vi "Check_Needed_Files.vi"(3 "error in":errorcluster, 6 "Data Cluster":T1 {"Shaft"."dmin" format="%#_7g"; "Shaft"."dmax" format="%#_7g"; "Shaft"."Fundamental Dev" format="%#_7g"; "Shaft"."Tolerance Grade (IT) Shaft" format="%#_7g"; "Hole"."Dmin" format="%#_7g"; "Hole"."Tolerance Grade (IT)" format="%#_7g"}) -> (0 "error out 2":errorcluster)   [LabVIEW 2023]
uses:
  TypeDef/Data_Cluster.ctl
  <vilib>/MGI/Panel Manager/Panel/Panel/Window/Window.lvclass
  C:/Program Files (x86)/National Instruments/LabVIEW 2023/vi.lib/MGI/Panel Manager/Panel/Panel/Panel.lvclass
  TypeDef/Units.ctl
  TypeDef/Method_Info.ctl
  TypeDef/Hole_Data.ctl
  TypeDef/Shaft_Data.ctl
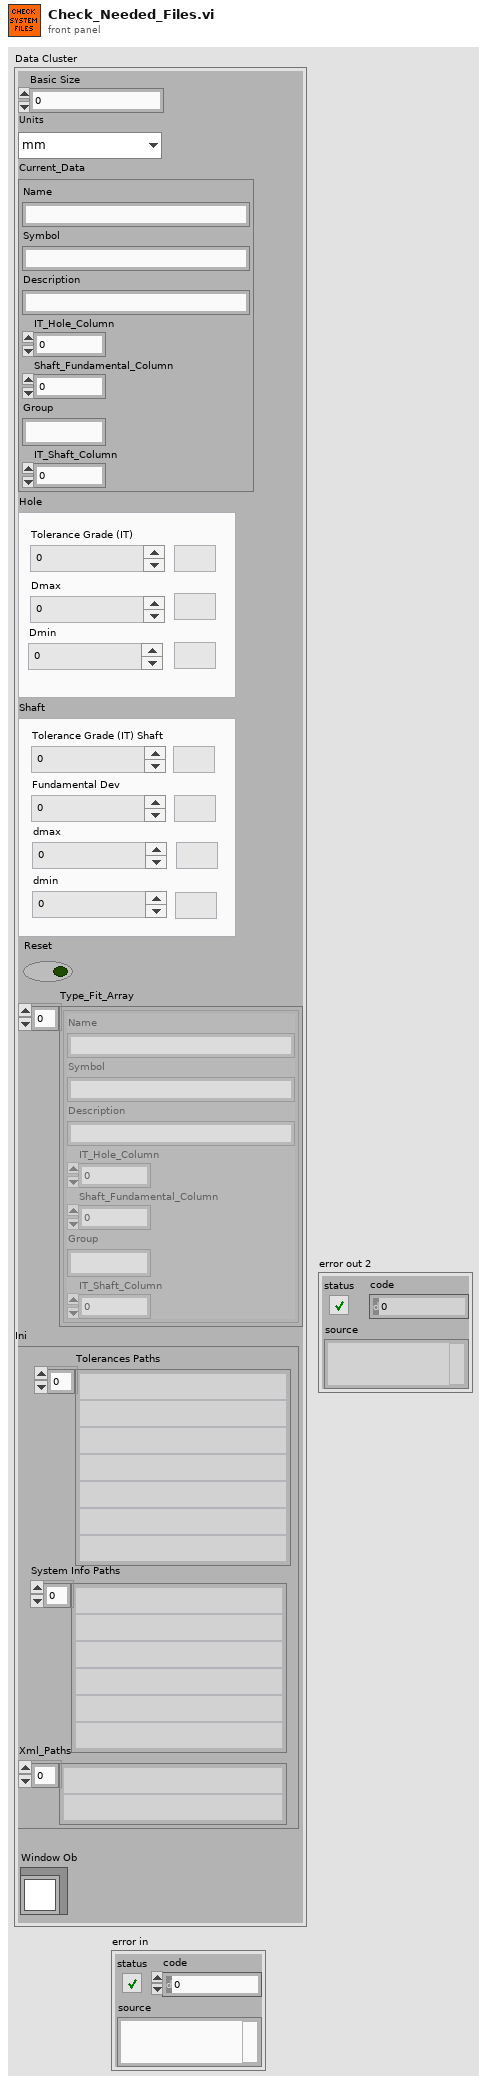
[diagram p1: front panel]
types:
  T1 = typedef "Data_Cluster.ctl" = cluster{"Basic Size ":dbl, "Units":T2, "Current_Data":T3, "Hole":T4, "Shaft":T5, "Reset":bool, "Type_Fit_Array":T3[], "Ini":cluster{"Tolerances Paths":path[], "System Info Paths":path[], "Xml_Paths":path[]}, "Window Ob":refnum<class "Window.lvclass">}
  T2 = typedef "Units.ctl" = enum16{"mm", "in"}
  T3 = typedef "Method_Info.ctl" = cluster{"Name":string, "Symbol":string, "Description":string, "IT_Hole_Column":i32, "Shaft_Fundamental_Column":i32, "Group":string, "IT_Shaft_Column":i32}
  T4 = typedef "Hole_Data.ctl" = cluster{"Tolerance Grade (IT)":dbl, "Dmax":dbl, "Units Hole":cluster{"units_it":string, "units_Dmax\nUnits_Dmax":string, "Units_Dmin":string}, "Dmin":dbl}
  T5 = typedef "Shaft_Data.ctl" = cluster{"Tolerance Grade (IT) Shaft":dbl, "Units Shaft":cluster{"Units_FundamentalDev":string, "Units_dmax":string, "Units_dmin":string, "Units_IT_Shaft":string}, "Fundamental Dev":dbl, "dmax":dbl, "dmin":dbl}
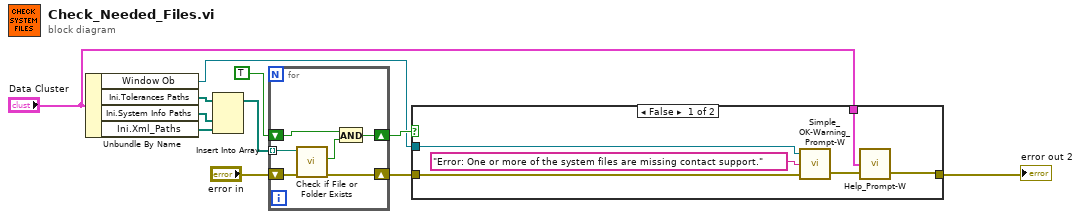
[diagram p0: block diagram]
diagram:
  n1 = Unbundle By Name("Data Cluster") -> ("Window Ob"=w3:refnum<class "Window.lvclass">, "Ini.Tolerances Paths"=w10:path[], "Ini.System Info Paths"=w9:path[], "Ini.Xml_Paths"=w8:path[])
  n2 = Insert Into Array(array=w10, new element #1=w9, new element #2=w8) -> (w7:path[])  [unwired: 1 in]
  n3 = for {
    shift-right: [w12] -> w4
    shift-left: "error in" -> [w17]
    shift-right: [w15] -> w6
    shift-left: TRUE -> [w16]
    tunnel: w7 -> [w13] mode=indexing
    n4 = call <vilib>:"Check if File or Folder Exists.vi"("error in (no error)"=w17, "path"=w13) -> ("error out"=w12:errorcluster, "file or folder exists?"=w14:bool)  [unwired: 7 in, 1 out]
    n5 = And(x=w16, y=w14) -> (x .and. y?=w15:bool)
  }
  n6 = case shown="False" w6 {
    tunnel: w4 -> [w23 w24]
    tunnel: w3 -> [w22 _]
    tunnel: [w19 w24] -> w2
    tunnel: "Data Cluster" -> [w18 _]
    frame False {
      n7 = call "Simple_OK-Warning_Prompt-W.vi"("error in"=w23, "User Message In"="Error: One or more of the system files are missing contact support.", "Panel In"=w22) -> ("error out"=w20:errorcluster)  [unwired: 1 in, 1 out]
      n8 = call "Help_Prompt-W.vi"("error in (no error)"=w20, "Data Cluster"=w18) -> ("error out"=w19:errorcluster)  [unwired: 2 in]
    }
    frame True {
    }
  }
  "error out 2" <- w2
